vi "Current VIs Parents Ref.vi"() -> (1 "Calling VI's Reference":refnum<vi>)   [LabVIEW 2012, in "VIRef.lvlib"]
doc: "Gets a reference to the parent of the VI calling this function. This is useful for creating reusable VIs that opperate on their parent.\n\n<b>Note:</b> The <b>Calling VI's Reference</b> should be closed, when finished with."
uses:
  VIRef.lvlib
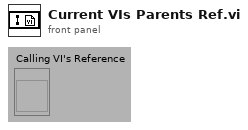
[diagram p1: front panel]
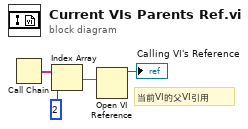
[diagram p0: block diagram]
diagram:
  # "当前VI的父VI引用"
  n1 = Call Chain() -> (call chain=w4:string[])
  n2 = Index Array(array=w4, index=2 ("Index")) -> (element=w2:string)
  n3 = Open VI Reference(vi path=w2) -> (vi reference=→"Calling VI's Reference":refnum<vi>)  [unwired: 5 in, 1 out]
